vi "Cleanup.vi"(8 "error in (no error)":errorcluster, 11 "Linux System SAL in":refnum<class "Linux System SAL.lvclass">) -> (0 "error out":errorcluster)   [LabVIEW 2020, in "Volatus.lvlib" / "Linux System SAL.lvclass"]
uses:
  Linux System SAL.lvclass
  Linux System SAL.lvclass/Linux System SAL.ctl
  <vilib>/nisyscfg/nisyscfg.lvlib
  <vilib>/nisyscfg/Close (Hardware).vi
  <vilib>/nisyscfg/Close (System).vi
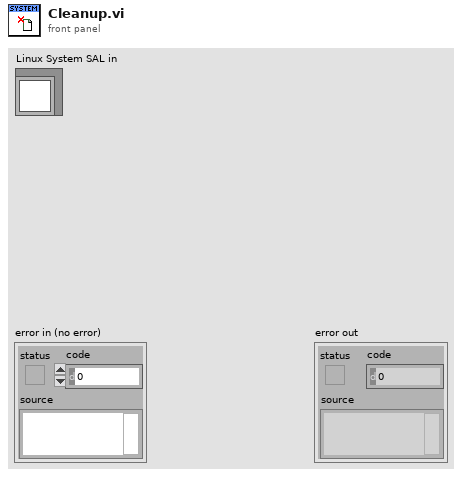
[diagram p1: front panel]
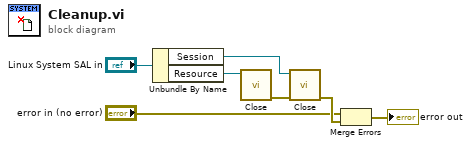
[diagram p0: block diagram]
diagram:
  n1 = Unbundle By Name("Linux System SAL in") -> ("Session"=w5:refnum<k21>, "Resource"=w6:refnum<k20>)
  n2 = call-poly <vilib>:"Close.vi"("Resource in"=w6) -> ("error out"=w7:errorcluster)  [unwired: 10 in]
  n3 = call-poly <vilib>:"Close.vi"("error in (no error)"=w7, "Session in"=w5) -> ("error out"=w4:errorcluster)  [unwired: 9 in]
  n4 = Merge Errors("error in (no error)", w4) -> (→"error out":errorcluster)
